vi "[GV]_Protocol String Send.vi"() -> ()   [LabVIEW 2016]
panel:
  out "Protocol String Send":string
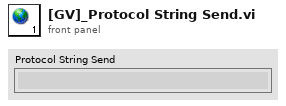
[diagram p1: front panel]
diagram:
